vi "Read_SetTestInformaton.vi"(8 "error in (no error)":errorcluster caption="错误输入（无错误）") -> (0 "error out":errorcluster caption="错误输出", 1 "数组 2":string[](array[string]), 2 "appended path":path, 3 "引用句柄输出":T1 caption="refnum out", 4 "数组":string[](array[string]))   [LabVIEW 2018]
uses:
  <vilib>/Utility/config.llb/Config Data RefNum.ctl
  Global.vi
  <vilib>/Utility/config.llb/Read Key (String).vi
  <vilib>/Utility/config.llb/NI_LVConfig.lvlib
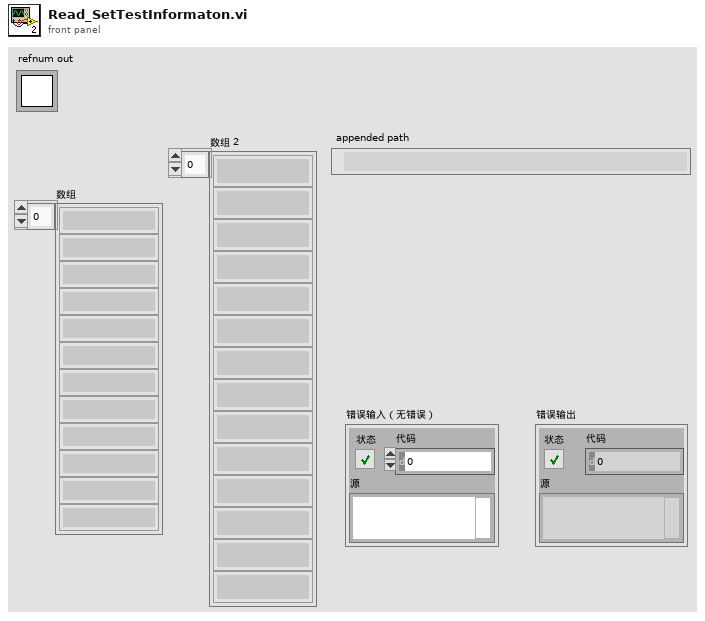
[diagram p1: front panel]
types:
  T1 = typedef "NI_LVConfig.lvlib/Config Data RefNum.ctl" = refnum<k1>
  T2 = enum32{"invalid app kind", "Development System", "Run Time System", "Student Edition", "Embedded LabVIEW", "Evaluation", "Custom"}
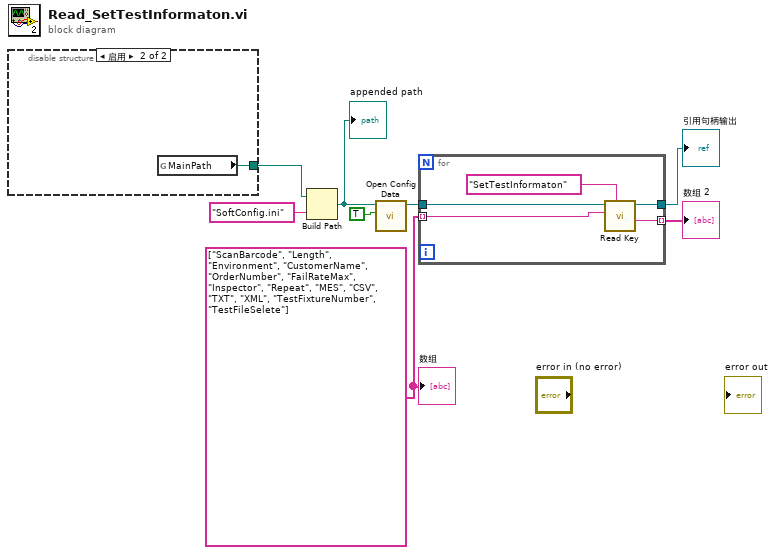
[diagram p0: block diagram]
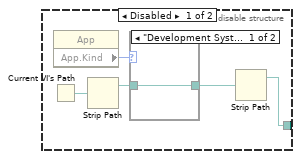
[diagram p2: hidden frame]
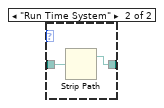
[diagram p3: hidden frame]
diagram:
  w8 = string[] ["ScanBarcode", "Length", "Environment", "CustomerName", "OrderNumber", "FailRateMax", "Inspector", "Repeat", "MES", "CSV", "TXT", "XML", "TestFixtureNumber", "TestFileSelete"]
  n1 = disable-structure shown="启用" {
    disable-tunnel: [w9 w17] -> w2
    frame Disabled {
      n2 = Current VI's Path() -> (path=w13:path)
      n3 = property class="App"() -> ("App.Kind"=w11:T2)  [unwired: 2 in, 2 out]
      n4 = Strip Path(path=w13) -> (stripped path=w12:path)  [unwired: 1 out]
      n5 = case shown="\"Development System\", 默认" w11 {
        tunnel: w12 -> [w14 w16]
        tunnel: [w14 w15] -> w10
        frame "Development System", Default {
        }
        frame "Run Time System" {
          n6 = Strip Path(path=w16) -> (stripped path=w15:path)  [unwired: 1 out]
        }
      }
      n7 = Strip Path(path=w10) -> (stripped path=w9:path)  [unwired: 1 out]
    }
    frame Enabled {
      n8 = global read "Global.vi" "MainPath"() -> (w17:path)
    }
  }
  n9 = Build Path(base path=w2, name or relative path="SoftConfig.ini" ("名称或相对路径")) -> (appended path=w3:path)
  "appended path" <- w3
  n10 = call <vilib>:"Open Config Data.vi"("create file if necessary (T)"=TRUE, "configuration file path"=w3) -> ("refnum"=w5:T1)  [unwired: 7 in, 2 out]
  n11 = for {
    tunnel: w8 -> [w22] mode=indexing
    tunnel: w5 -> [w21]
    tunnel: [w19] -> w7 mode=indexing
    tunnel: [w18] -> w6
    n12 = call-poly <vilib>:"Read Key.vi"("section"="SetTestInformaton", "key"=w22, "refnum"=w21) -> ("value"=w19:string, "refnum out"=w18:T1)  [unwired: 5 in, 2 out]
  }
  "数组 2" <- w7
  "引用句柄输出" <- w6
  "数组" <- w8
